vi "Create_New_Build.vi"(6 "buildSpecName":string, 7 "Programmatic? (false)":bool, 8 "error in (no error)":errorcluster, 9 "buildObject":T1, 10 "Destination Path":path, 11 "AB_DepDLL in":refnum<class "AB_DepDLL.lvclass">) -> (0 "error out":errorcluster, 3 "AB_DepDLL out":refnum<class "AB_DepDLL.lvclass">)   [LabVIEW 2020, in "AB_DepDLL.lvclass"]
uses:
  <vilib>/AppBuilder/AB_Classes/DepDLL/AB_DepDLL.lvclass
  e:/builds/penguin/labview/branches/2020/dev/dist/vi.lib/AppBuilder/AB_Classes/Build/AB_Build.lvclass
  e:/builds/penguin/labview/branches/2020/dev/dist/vi.lib/AppBuilder/AB_Classes/DLL/AB_DLL.lvclass
  <resource>/Framework/Providers/API/ItemRef.ctl
  <vilib>/AppBuilder/AB_Classes/DLL/AB_DLL.lvclass
  <vilib>/AppBuilder/AB_Classes/Deployment/AB_Deployment.lvlib
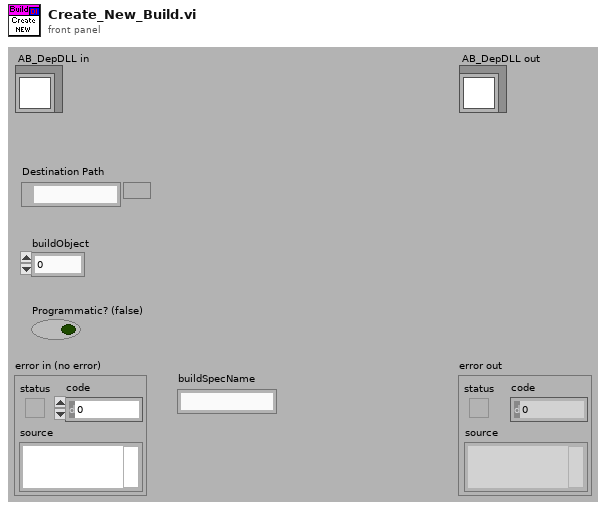
[diagram p1: front panel]
types:
  T1 = typedef "ItemRef.ctl" = u64
  T2 = typedef "AB_DLL.ctl" = cluster{"delayOSMsg":bool, "includeHeaders":bool, "embeddedRTE":bool, "headerGUID":string, "libGUID":string, "compatibilityWith2011":bool, "includeTypeLibrary":bool, "privateExecutionSystem":bool}
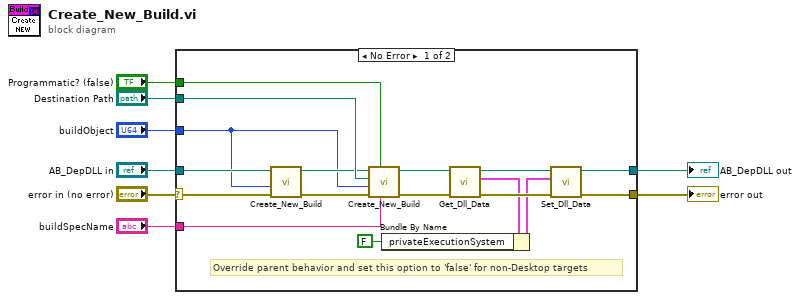
[diagram p0: block diagram]
diagram:
  n1 = case shown="No Error" "error in (no error)" {
    selector: "error in (no error)" -> [w20 w26]
    tunnel: "buildSpecName" -> [w25 _]
    tunnel: "Programmatic? (false)" -> [w24 _]
    tunnel: "buildObject" -> [w18 _]
    tunnel: "Destination Path" -> [w23 _]
    tunnel: "AB_DepDLL in" -> [w22 w27]
    tunnel: [w12 w26] -> w3
    tunnel: [w15 w27] -> w2
    frame No Error {
      # "Override parent behavior and set this option to 'false' for non-Desktop targets"
      n2 = call <vilib>:"Create_New_Build.vi"("error in (no error)"=w20, "buildObject"=w18, "Build in"=w22) -> ("error out"=w19:errorcluster, "Build out"=w21:refnum<class "AB_DepDLL.lvclass">)  [unwired: 7 in]
      n3 = call-parent <vilib>:"Create_New_Build.vi"("buildSpecName"=w25, "Programmatic? (false)"=w24, "error in (no error)"=w19, "buildObject"=w18, "Destination Path"=w23, "AB_DLL in"=w21) -> ("error out"=w13:errorcluster, "AB_DLL out"=w16:refnum<class "AB_DepDLL.lvclass">)  [unwired: 4 in]
      n4 = call <vilib>:"Get_Dll_Data.vi"("error in (no error)"=w13, "Class in"=w16) -> ("error out"=w14:errorcluster, "data"=w11:T2, "Class out"=w17:refnum<class "AB_DepDLL.lvclass">)  [unwired: 7 in]
      n5 = Bundle By Name(cluster=w11, "privateExecutionSystem"=FALSE) -> (w10:T2)
      n6 = call <vilib>:"Set_Dll_Data.vi"("error in (no error)"=w14, "data"=w10, "Class in"=w17) -> ("error out"=w12:errorcluster, "Class out"=w15:refnum<class "AB_DepDLL.lvclass">)  [unwired: 7 in]
    }
    frame Error {
    }
  }
  "error out" <- w3
  "AB_DepDLL out" <- w2
